vi "Build Time Stamp Message.vi"() -> (3 "Array":u32[](array[numeric]) format="%.0x")   [LabVIEW 2014]
panel:
  out "remaining string":string
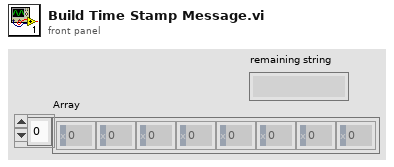
[diagram p1: front panel]
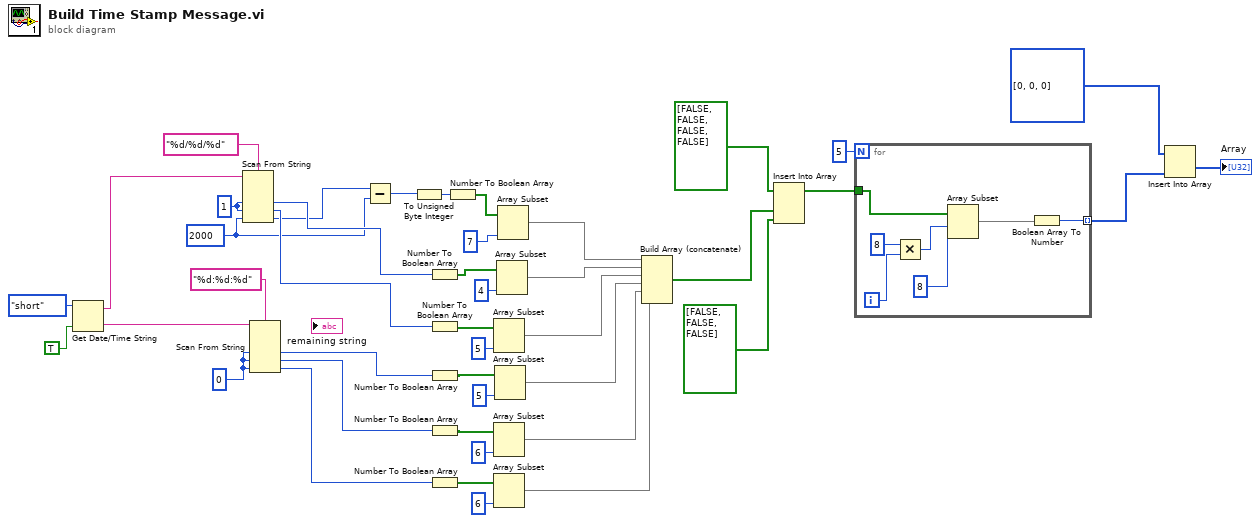
[diagram p0: block diagram]
diagram:
  w7 = u8 0 ("default value 3")
  w4 = 2000 ("default value 3")
  w13 = u8 1 ("default value 1")
  n1 = Get Date/Time String(date format (0)=enum16{"short", "long", "abbreviated"}."short", want seconds? (F)=TRUE) -> (date string=w2:string, time string=w3:string)  [unwired: 1 in]
  n2 = Scan From String(format string="%d/%d/%d", input string=w2, default 1=w13, default 2=w13, default 3=w4) -> (output 1=w12:u8, output 2=w11:u8, output 3=w5:i32)  [unwired: 2 in, 3 out]
  n3 = Scan From String(format string="%d:%d:%d", input string=w3, default 1=w7, default 2=w7, default 3=w7) -> (output 1=w1:u8, output 2=w9:u8, output 3=w8:u8)  [unwired: 2 in, 3 out]
  n4 = Subtract(x=w5, y=w4) -> (x-y=w6:i32)
  n5 = To Unsigned Byte Integer(number=w6) -> (unsigned 8bit integer=w25:u8)
  n6 = Number To Boolean Array(number=w12) -> (Boolean array=w42:bool[])
  n7 = Number To Boolean Array(number=w11) -> (Boolean array=w39:bool[])
  n8 = Number To Boolean Array(number=w1) -> (Boolean array=w37:bool[])
  n9 = Number To Boolean Array(number=w9) -> (Boolean array=w35:bool[])
  n10 = Number To Boolean Array(number=w8) -> (Boolean array=w33:bool[])
  n11 = Number To Boolean Array(number=w25) -> (Boolean array=w26:bool[])
  n12 = Array Subset(array=w39, length=5) -> (w30:bool[])  [unwired: 1 in]
  n13 = Array Subset(array=w35, length=6) -> (w28:bool[])  [unwired: 1 in]
  n14 = Array Subset(array=w33, length=6) -> (w27:bool[])  [unwired: 1 in]
  n15 = Array Subset(array=w37, length=5) -> (w29:bool[])  [unwired: 1 in]
  n16 = Array Subset(array=w42, length=4) -> (w31:bool[])  [unwired: 1 in]
  n17 = Array Subset(array=w26, length=7) -> (w32:bool[])  [unwired: 1 in]
  n18 = Build Array (concatenate)(w32, w31, w30, w29, w28, w27) -> (w24:bool[])
  n19 = Insert Into Array(array=bool[] [FALSE, FALSE, FALSE, FALSE], new element #1=w24, new element #2=bool[] [FALSE, FALSE, FALSE] ("array")) -> (w21:bool[])  [unwired: 1 in]
  n20 = for {
    N: 5 -> [_]
    tunnel: w21 -> [w49]
    tunnel: [w44] -> w19 mode=indexing
    i -> [w46]
    n21 = Multiply(x=8, y=w46) -> (x*y=w48:i32)
    n22 = Array Subset(array=w49, index=w48, length=8) -> (w50:bool[])
    n23 = Boolean Array To Number(Boolean array=w50) -> (number=w44:u32)
  }
  n24 = Insert Into Array(array=u32[] [0, 0, 0] ("Array 2"), new element=w19) -> (→"Array":u32[])  [unwired: 1 in]
